vi "Close Data Logging Manager Reference.vi"(8 "error in (no error)":errorcluster, 11 "Data Logging Manager Ref in":T1) -> (0 "error out":errorcluster)   [LabVIEW 2020, in "NI_VS Data Logging API.lvlib"]
doc: "Closes the connection to the data logging service on the VeriStand Gateway."
uses:
  <vilib>/NI VeriStand/Execution/DataLogging/NI_VS Data Logging API.lvlib
  <vilib>/NI VeriStand/Execution/DataLogging/IDataLogging Ref.ctl
  NationalInstruments.VeriStand.ClientAPI
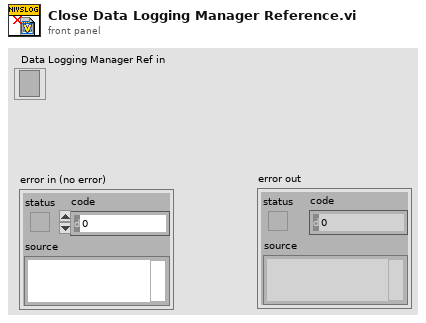
[diagram p1: front panel]
types:
  T1 = typedef "NI_VS Data Logging API.lvlib/IDataLogging Ref.ctl" = refnum<k24>
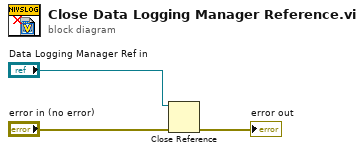
[diagram p0: block diagram]
diagram:
  n1 = Close Reference(reference="Data Logging Manager Ref in", error in (no error)="error in (no error)") -> (error out=→"error out":errorcluster)
